vi "Untitled 1.vi"() -> ()   [LabVIEW 2011]
uses:
  <vilib>/express/express arith-compare/Formula/XNode/ExpressFormulaBlockNode.xnode
panel:
  out "numero":dbl
  out "pomedio":dbl
  out "contador":dbl
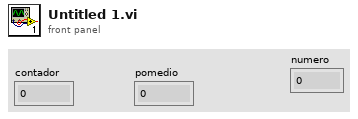
[diagram p1: front panel]
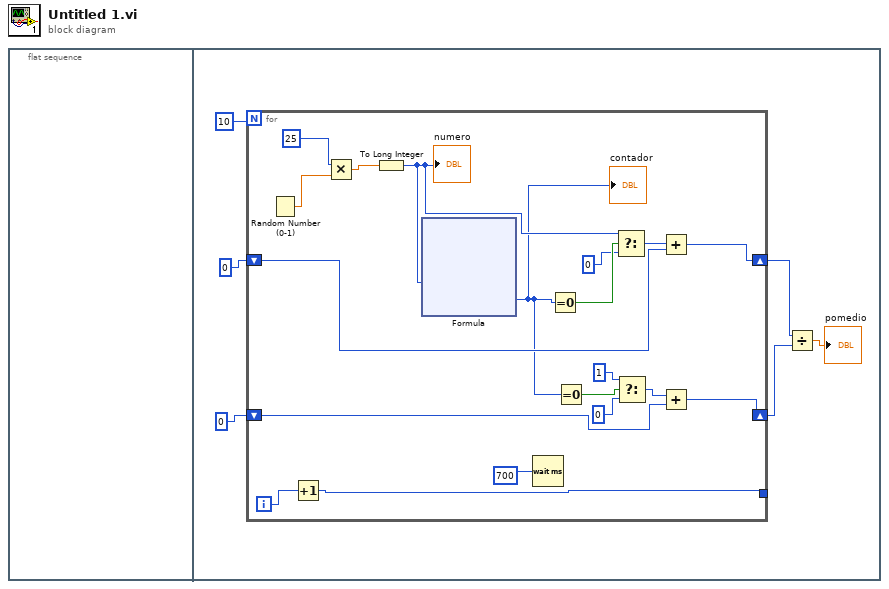
[diagram p0: block diagram]
diagram:
  n1 = flat-sequence {
    frame #0 {
    }
    frame #1 {
      n2 = for {
        N: 10 -> [_]
        shift-right: [w18] -> w2
        shift-left: 0 -> [w19]
        shift-right: [w11] -> w3
        shift-left: 0 -> [w12]
        tunnel: [w7] -> _
        i -> [w8]
        n3 = Random Number (0-1)() -> (number: 0 to 1=w23:dbl)
        n4 = Increment(x=w8) -> (x+1=w7:i32)
        n5 = Multiply(x=25, y=w23) -> (x*y=w25:dbl)
        n6 = To Long Integer(number=w25) -> (32bit integer=w17:i32)
        "numero" <- w17
        n7 = xnode "Formula"("X1"=w17) -> ("Result"=w9:i32)  [unwired: 1 in, 1 out]
        "contador" <- w9
        n8 = Wait (ms)(milliseconds to wait=700) -> ()  [unwired: 1 out]
        n9 = Equal To 0?(x=w9) -> (x = 0?=w22:bool)
        n10 = Equal To 0?(x=w9) -> (x = 0?=w16:bool)
        n11 = Select(t=w17, s=w22, f=0) -> (s? t:f=w20:i32)
        n12 = Select(t=1, s=w16, f=0) -> (s? t:f=w13:i32)
        n13 = Add(x=w20, y=w19) -> (x+y=w18:i32)
        n14 = Add(x=w13, y=w12) -> (x+y=w11:i32)
      }
      n15 = Divide(x=w2, y=w3) -> (x/y=→"pomedio":dbl)
    }
  }
